vi "DSF.Engine.Memory.ObjectPool.Bundle.Create.vi"(8 "error in (no error)":errorcluster, 10 "index":i32, 11 "Object":refnum<class>) -> (0 "error out":errorcluster, 3 "ObjectPool Bundle":refnum<class "DSF.Engine.Memory.ObjectPool.Bundle.lvclass">)   [LabVIEW 2016, in "DSF.Engine.lvlib" / "DSF.Engine.Memory.ObjectPool.Bundle.lvclass"]
uses:
  DSF.Engine.Memory.ObjectPool.Bundle.lvclass
  DSF.Engine.Memory.ObjectPool.Bundle.lvclass/DSF.Engine.Memory.ObjectPool.Bundle.ctl
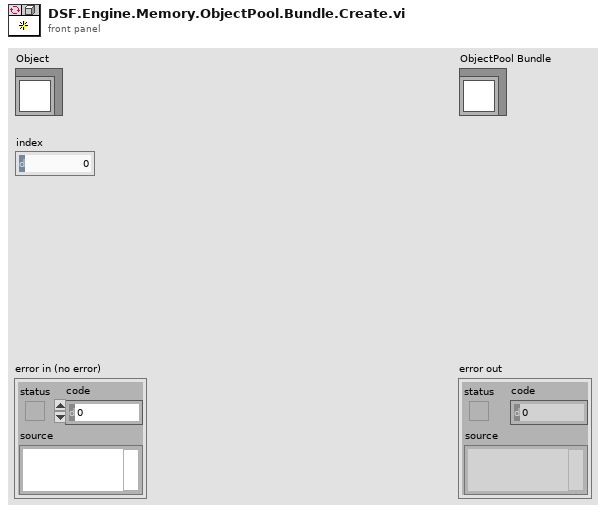
[diagram p1: front panel]
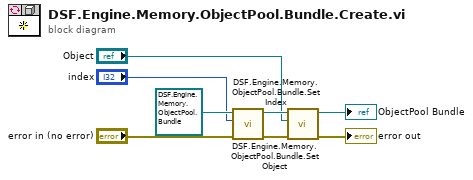
[diagram p0: block diagram]
diagram:
  n1 = call "DSF.Engine.Memory.ObjectPool.Bundle.Set Index.vi"("error in (no error)"="error in (no error)", "Index"="index", "ObjectPool Bundle in"=refnum<class "DSF.Engine.Memory.ObjectPool.Bundle.lvclass"> refnum) -> ("error out"=w5:errorcluster, "ObjectPool Bundle out"=w6:refnum<class "DSF.Engine.Memory.ObjectPool.Bundle.lvclass">)  [unwired: 7 in]
  n2 = call "DSF.Engine.Memory.ObjectPool.Bundle.Set Object.vi"("error in (no error)"=w5, "Object"="Object", "ObjectPool Bundle in"=w6) -> ("error out"=→"error out":errorcluster, "ObjectPool Bundle out"=→"ObjectPool Bundle":refnum<class "DSF.Engine.Memory.ObjectPool.Bundle.lvclass">)  [unwired: 7 in]
